vi "SetBuzzerFrequency.vi"(10 "error in (no error)":errorcluster, 11 "Frequency":u16(knob) scale=0.0..10000.0) -> (3 "error out":errorcluster)   [LabVIEW 2013]
uses:
  <vilib>/myRIO/Instrument Drivers/Onboard IO/I2C/vis/Smart Open.vi
  <vilib>/myRIO/Instrument Drivers/Onboard IO/I2C/vis/Configure.vi
  <vilib>/myRIO/Instrument Drivers/Onboard IO/I2C/vis/Write Read.vi
  <vilib>/myRIO/Instrument Drivers/Onboard IO/I2C/vis/Open.vi
  <vilib>/myRIO/Common/Instrument Driver Framework/myRIO v1.0/I2C/vis/myRIO v1.1 Open I2C.vi
  <vilib>/myRIO/Common/Instrument Driver Framework/Utilities/vis/Validate Channels.vi
  <vilib>/myRIO/Common/Instrument Driver Framework/myRIO v1.0/I2C/vis/myRIO v1.0 Reserve I2C.vi
  <vilib>/myRIO/Common/Instrument Driver Framework/myRIO v1.0/I2C/vis/myRIO v1.0 Build MUX Configuration I2C.vi
  <vilib>/myRIO/Common/Instrument Driver Framework/myRIO v1.0/Resource Manager/vis/myRIO v1.0 Reserve Channel List.vi
  <vilib>/myRIO/Common/Instrument Driver Framework/myRIO v1.0/Resource Manager/vis/myRIO v1.0 Create Configuration List.vi
  <vilib>/myRIO/Common/Instrument Driver Framework/myRIO v1.0/Resource Manager/vis/myRIO v1.0 Reserve Channel.vi
  <vilib>/myRIO/Common/Instrument Driver Framework/myRIO v1.0/Resource Manager/vis/myRIO v1.0 Unreserve Channel.vi
  <vilib>/myRIO/Common/Instrument Driver Framework/myRIO v1.0/Resource Manager/vis/myRIO v1.0 Build Mutex Name.vi
  <vilib>/myRIO/Common/Instrument Driver Framework/myRIO v1.0/myRIO v1.1 Open.vi
  <vilib>/Utility/VariantDataType/GetNumericInfo.vi
  <vilib>/Utility/error.llb/Error Cluster From Error Code.vi
  <vilib>/myRIO/Common/Instrument Driver Framework/Utilities/vis/IO Manager.vi
  <vilib>/myRIO/Common/Instrument Driver Framework/Utilities/vis/Configuration Manager.vi
  <vilib>/myRIO/Common/Instrument Driver Framework/myRIO v1.0/Resource Manager/vis/myRIO v1.0 Configure IO.vi
  <vilib>/myRIO/Common/Instrument Driver Framework/myRIO v1.0/myRIO v1.0 Close.vi
  <vilib>/myRIO/Common/Instrument Driver Framework/myRIO v1.0/I2C/vis/myRIO v1.0 Configure I2C.vi
  <vilib>/myRIO/Common/Instrument Driver Framework/myRIO v1.0/I2C/vis/myRIO v1.0 Write I2C.vi
  <vilib>/myRIO/Common/Instrument Driver Framework/myRIO v1.0/I2C/vis/myRIO v1.0 Read I2C.vi
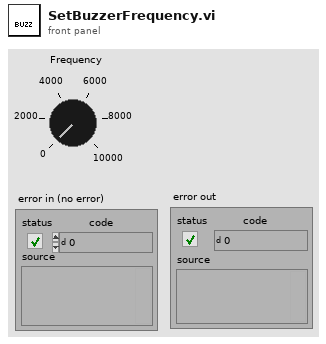
[diagram p1: front panel]
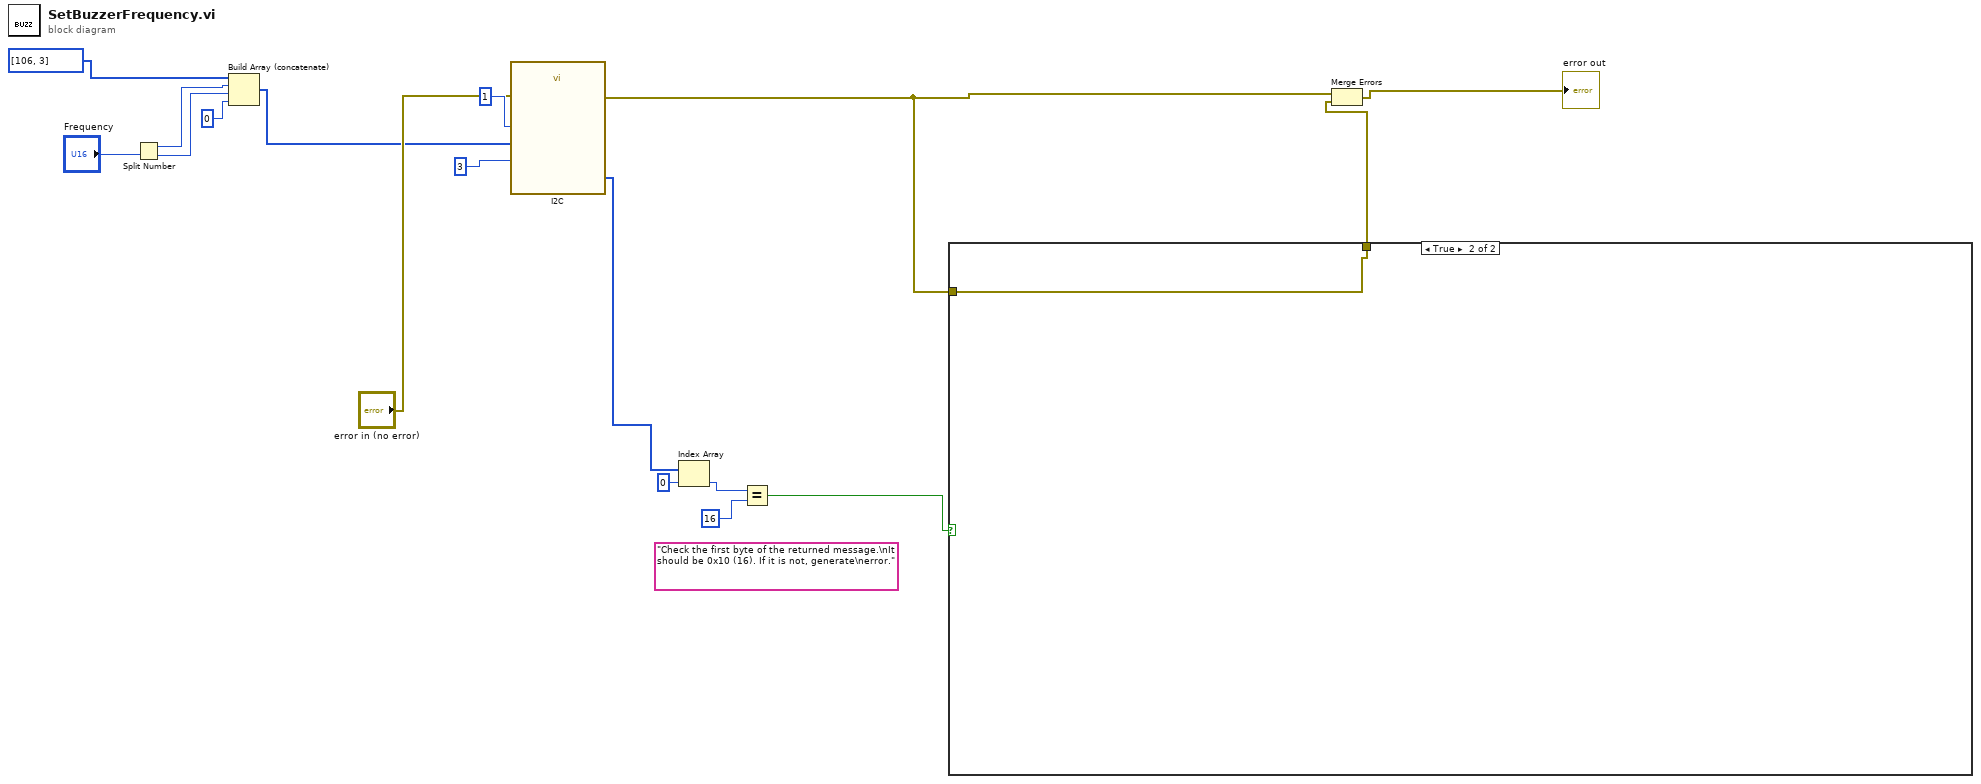
[diagram p0: block diagram]
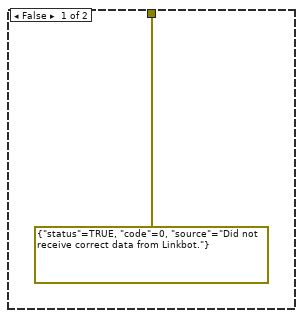
[diagram p2: hidden frame]
diagram:
  (unwired) "Check the first byte of the returned message.\nIt should be 0x10 (16). If it is not, generate\nerror."
  n1 = Split Number(x="Frequency") -> (hi(x)=w4:u8, lo(x)=w3:u8)
  n2 = Build Array (concatenate)(u8[] [106, 3], w4, w3, u8 0 ("element")) -> (w2:u8[])
  n3 = call "I2C"("Slave Address (7-bit)"=1, "Bytes to Write"=w2, "Byte Count"=3, "error in (no error)"="error in (no error)") -> ("Bytes Read"=w13:u8[], "error out"=w7:errorcluster)  [unwired: 22 in]
  n4 = Index Array(array=w13, index=0) -> (element=w11:u8)
  n5 = Equal?(x=w11, y=u8 16) -> (x = y?=w9:bool)
  n6 = case shown="True" w9 {
    tunnel: [errorcluster {"status"=TRUE, "code"=0, "source"="Did not receive correct data from Linkbot."} ("error constant") w19] -> w8
    tunnel: w7 -> [_ w19]
    frame False {
    }
    frame True {
    }
  }
  n7 = Merge Errors(w7, w8) -> (→"error out":errorcluster)
